vi "LWXPS_ZygoReadWord.vi"(0 "XPS Reference IN":refnum<k24>, 5 "Axis number":string, 7 "Register value":string, 11 "LabVIEW error IN":errorcluster) -> (4 "XPS Reference OUT":refnum<k24>, 6 "Returned error code":i32, 8 "Response":string, 10 "XPS Error String":string, 15 "LabVIEW error OUT":errorcluster)   [LabVIEW 2014]
uses:
  D:/XPSQ8_LabView_Library/Development/Source/Dll/Newport.XPS.CommandInterface.dll
  Dll/Newport.XPS.CommandInterface.dll
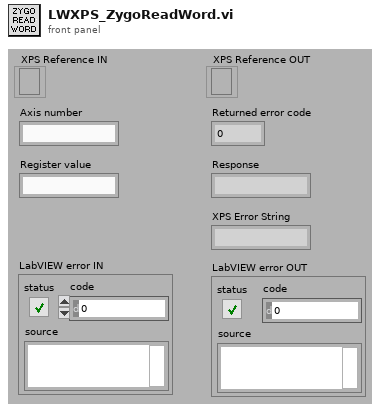
[diagram p1: front panel]
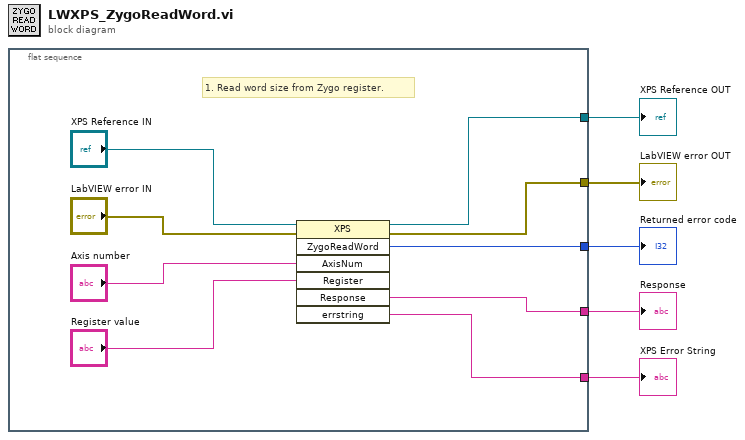
[diagram p0: block diagram]
diagram:
  n1 = flat-sequence {
    tunnel: [w12] -> w5
    tunnel: [w9] -> w4
    tunnel: [w13] -> w3
    tunnel: [w6] -> w2
    tunnel: [w8] -> w1
    frame #0 {
      # "1. Read word size from Zygo register."
      n2 = invoke class="XPS" method="ZygoReadWord"(reference="XPS Reference IN", error in="LabVIEW error IN", "AxisNum"="Axis number", "Register"="Register value") -> (reference out=w12:refnum<k24>, error out=w9:errorcluster, "ZygoReadWord"=w13:i32, "Response"=w8:string, "errstring"=w6:string)  [unwired: 3 in, 2 out]
    }
  }
  "XPS Reference OUT" <- w5
  "LabVIEW error OUT" <- w4
  "Returned error code" <- w3
  "XPS Error String" <- w2
  "Response" <- w1
